vi "solar Exit (Children).vi"(8 "error in (no error)":errorcluster, 11 "solar in":refnum<class "solar.lvclass">) -> (0 "error out":errorcluster, 3 "solar out":refnum<class "solar.lvclass">)   [LabVIEW 2018]
doc: "If this is the top level main target, this enqueues the 'EXIT' command to all child targets."
uses:
  solar.lvclass
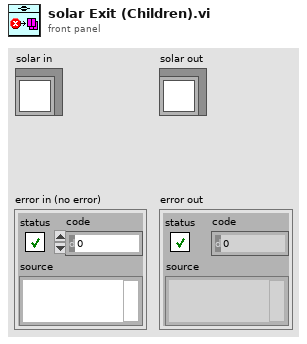
[diagram p1: front panel]
types:
  T1 = typedef "solar_ctl Target Global.ctl" = cluster{"Target":string, "Q":refnum<queue>, "UE":refnum<user-event>, "VI":refnum<vi>, "Menu":refnum<k9>, "Data":refnum<data-value>, "Attributes":variant}
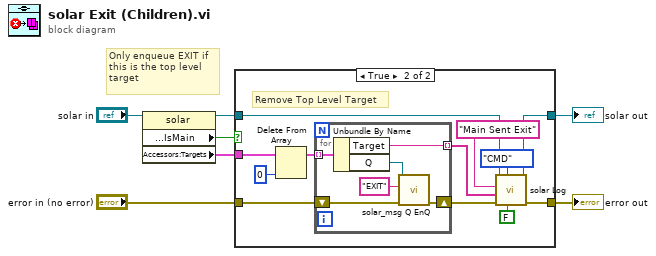
[diagram p0: block diagram]
diagram:
  # "Only enqueue EXIT if\nthis is the top level\ntarget"
  n1 = property class="solar"(reference="solar in") -> (reference out=w1:refnum<class "solar.lvclass">, "Accessors:Main.IsMain"=w5:bool, "Accessors:Targets"=w4:T1[])  [unwired: 1 in, 1 out]
  n2 = case shown="True" w5 {
    tunnel: "error in (no error)" -> [w9 w19]
    tunnel: [w9 w16] -> w7
    tunnel: w4 -> [_ w18]
    tunnel: [w8 w14] -> w2
    tunnel: w1 -> [w8 w15]
    frame False {
    }
    frame True {
      # "Remove Top Level Target"
      n3 = Delete From Array(array=w18, index=0) -> (array with subset deleted=w20:T1[])  [unwired: 1 in, 1 out]
      n4 = for {
        tunnel: w20 -> [w25] mode=indexing
        shift-right: [w26] -> w17
        shift-left: w19 -> [w27]
        tunnel: [w22] -> w13 mode=indexing
        n5 = Unbundle By Name(w25) -> ("Target"=w22:string, "Q"=w23:refnum<queue>)
        n6 = call "solar_msg Q EnQ.vi"("error in (no error)"=w27, "CMD (Last)"="EXIT" ("Packet"), "Queue in"=w23) -> ("error out"=w26:errorcluster)  [unwired: 6 in, 2 out]
      }
      n7 = call "solar Log.vi"("Clear Error? (T)"=FALSE, "Type (TLM)"=enum8{"CMD", "TLM"}."CMD", "error in (no error)"=w17, "DATA"=w13, "MSG"="Main Sent Exit", "solar in"=w15) -> ("error out"=w16:errorcluster, "solar out"=w14:refnum<class "solar.lvclass">)  [unwired: 4 in]
    }
  }
  "error out" <- w7
  "solar out" <- w2
